vi "(SubVI) Get Real Position to Deal with Stage Offset_YCC.vi"(4 "Axis":i32) -> (0 "Expect - Real move (nm)\nStage Offset\n+=more move\n-=less move":dbl, 1 "Real Current Commanded position (um)":dbl format="%0.5f")   [LabVIEW 2014]
uses:
  Main-Stage-PI/(Global) Current handle and LaserPower_YCC.vi
panel:
  out "second write":dbl
  out "precise current position (um)":dbl
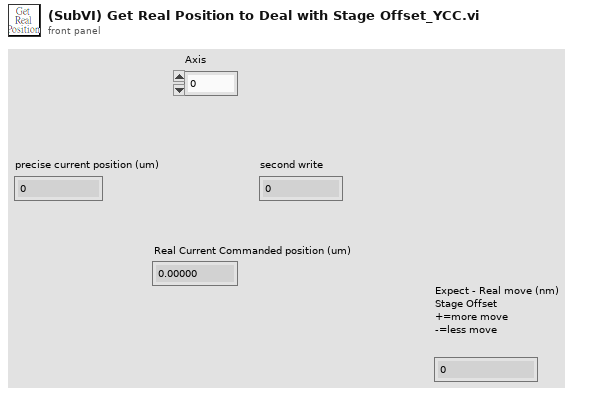
[diagram p1: front panel]
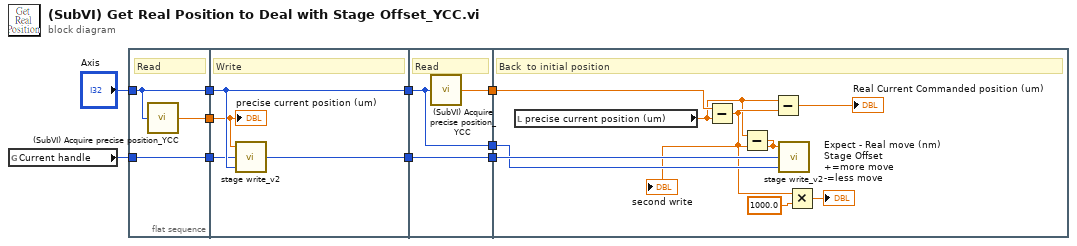
[diagram p0: block diagram]
diagram:
  n1 = global read "(Global) Current handle and LaserPower_YCC.vi" "Current handle"() -> (w6:i32)
  n2 = flat-sequence {
    tunnel: "Axis" -> [w12]
    tunnel: [w13] -> w10
    tunnel: [w12] -> w9
    tunnel: w6 -> [w11]
    tunnel: [w11] -> w5
    tunnel: w10 -> [w14]
    tunnel: w9 -> [w17]
    tunnel: [w17] -> w8
    tunnel: w5 -> [w16]
    tunnel: [w15] -> w2
    tunnel: w8 -> [w18]
    tunnel: [w20] -> w4
    tunnel: [w19] -> w3
    tunnel: w2 -> [w19]
    tunnel: [w18] -> w1
    tunnel: w4 -> [w26]
    tunnel: w3 -> [w29]
    tunnel: w1 -> [w28]
    frame #0 {
      # "Read"
      n3 = call "(SubVI) Acquire precise position_YCC.vi"("Axis"=w12) -> ("precise current position (um)"=w13:dbl)  [unwired: 4 in]
    }
    frame #1 {
      # "Write"
      n4 = call "stage write_v2.vi"("axis"=w17, "Incoming Handle"=w16, "position"=w14) -> ("out handle"=w15:i32)  [unwired: 2 in]
      "precise current position (um)" <- w14
    }
    frame #2 {
      # "Read"
      n5 = call "(SubVI) Acquire precise position_YCC.vi"("Axis"=w18) -> ("precise current position (um)"=w20:dbl)  [unwired: 4 in]
    }
    frame #3 {
      # "Back  to initial position"
      n6 = local read "precise current position (um)"() -> (w21:dbl)
      n7 = Subtract(x=w26, y=w21) -> (x-y=w22:dbl)
      n8 = Subtract(x=w21, y=w22) -> (x-y=w27:dbl)
      "second write" <- w27
      n9 = Subtract(x=w21, y=w22) -> (x-y=→"Real Current Commanded position (um)":dbl)
      n10 = call "stage write_v2.vi"("axis"=w28, "Incoming Handle"=w29, "position"=w27) -> ()  [unwired: 2 in, 1 out]
      n11 = Multiply(x=w22, y=1000.0) -> (x*y=→"Expect - Real move (nm)\nStage Offset\n+=more move\n-=less move":dbl)
    }
  }
